vi "Get Object to File.vi"(4 "Version ID":string, 6 "Chunk size (kB)":i32=5120 min=5120, 8 "error in (no error)":errorcluster, 9 "File":path, 10 "Object Path":string, 11 "Bucket in":refnum<class "Bucket.lvclass">) -> (0 "error out":errorcluster, 3 "Bucket out":refnum<class "Bucket.lvclass">)   [LabVIEW 2015, in "NI_AWS_S3.lvlib" / "Bucket.lvclass"]
doc: "This operation <B>uploads an object from a file</B> to a bucket <B>in multiple parts</B>. You can <B>set Chunk size (kB) to limit memory usage</B> of the operation."
uses:
  Bucket.lvclass
  GET Object Request Parameters.ctl
  Core/Request Range.ctl
  Core/NI_AWS_Core.lvlib
  NI_AWS_S3.lvlib
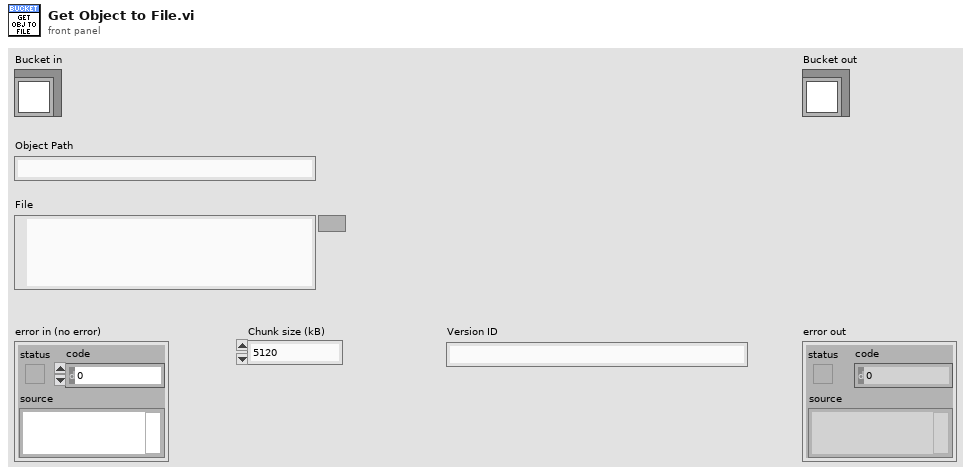
[diagram p1: front panel]
types:
  T1 = enum16{"open", "replace", "create", "open or create", "replace or create", "replace or create with confirmation"}
  T2 = typedef "NI_AWS_S3.lvlib/GET Object Request Parameters.ctl" = cluster{"Range":T3, "If Modified Since":timestamp, "If Unmodified Since":timestamp, "Matching ETag":string, "Nonmatching ETag":string}
  T3 = typedef "NI_AWS_Core.lvlib/Request Range.ctl" = cluster{"Start":i64, "Length":i64}
  T4 = typedef "NI_AWS_S3.lvlib/GET Object Result Parameters.ctl" = cluster{"Content Length (bytes)":u64, "Content Type":string, "ETag":string, "Delete Marker":bool, "Version ID":string, "Object Size (bytes)":u64}
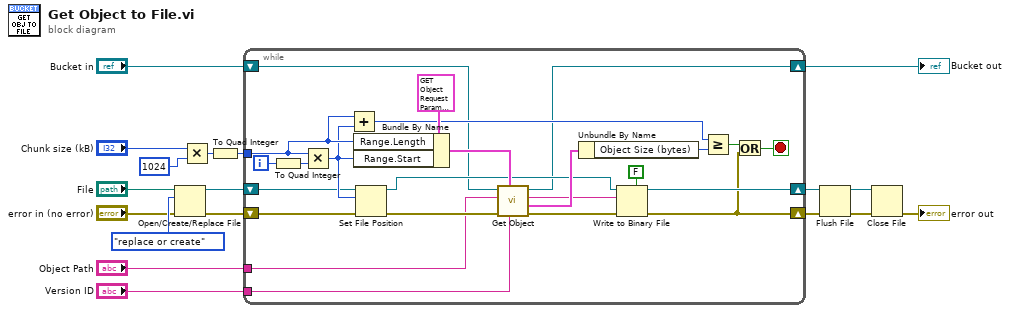
[diagram p0: block diagram]
diagram:
  n1 = Open/Create/Replace File(file path (use dialog)="File", error in="error in (no error)", operation (0:open)=T1."replace or create") -> (refnum out=w17:refnum<file>, error out=w16:errorcluster)  [unwired: 3 in, 1 out]
  n2 = Multiply(x="Chunk size (kB)", y=1024) -> (x*y=w10:i32)
  n3 = To Quad Integer(1:w10) -> (0:w9:i64)
  n4 = while {
    tunnel: w9 -> [w27]
    shift-right: [w31] -> w14
    shift-left: w17 -> [w25]
    shift-right: [w21] -> w15
    shift-left: w16 -> [w36]
    shift-right: [w24] -> w6
    shift-left: "Bucket in" -> [w23]
    tunnel: "Object Path" -> [w20]
    tunnel: "Version ID" -> [w19]
    i -> [w29]
    stop <- w22 stop-if-true
    n5 = To Quad Integer(1:w29) -> (0:w28:i64)
    n6 = Multiply(x=w27, y=w28) -> (x*y=w26:i64)
    n7 = Add(x=w27, y=w26) -> (x+y=w38:i64)
    n8 = Bundle By Name(cluster=T2 {"Range"={"Start"=0, "Length"=0}, "If Modified Since"=timestamp(0 s since 1904-01-01), "If Unmodified Since"=timestamp(0 s since 1904-01-01), "Matching ETag"="", "Nonmatching ETag"=""} ("Request Parameters"), "Range.Length"=w27, "Range.Start"=w26) -> (w41:T2)
    n9 = Set File Position(offset (in bytes) (0)=w26, refnum=w25, error in=w36) -> (refnum out=w32:refnum<file>, error out=w35:errorcluster)  [unwired: 1 in]
    n10 = call "Get Object.vi"("Version ID"=w19, "Request Parameters"=w41, "error in (no error)"=w35, "Object Path"=w20, "Bucket in"=w23) -> ("error out"=w34:errorcluster, "Object Info"=w40:T4, "Data"=w33:string, "Bucket out"=w24:refnum<class "Bucket.lvclass">)  [unwired: 2 in, 1 out]
    n11 = Unbundle By Name(w40) -> ("Object Size (bytes)"=w39:u64)
    n12 = Write to Binary File(file (use dialog)=w32, data=w33, error in=w34, 5:FALSE ("prepend array or string size? (T)")) -> (refnum out=w31:refnum<file>, error out=w21:errorcluster)  [unwired: 2 in, 1 out]
    n13 = Greater Or Equal?(x=w38, y=w39) -> (x >= y?=w37:bool)
    n14 = Or(x=w37, y=w21) -> (x .or. y?=w22:bool)
  }
  "Bucket out" <- w6
  n15 = Flush File(refnum=w14, error in=w15) -> (refnum out=w12:refnum<file>, error out=w13:errorcluster)
  n16 = Close File(refnum=w12, error in=w13) -> (error out=→"error out":errorcluster)  [unwired: 1 out]
